vi "xijk_array_to_queue_end.vi"(8 "error in":errorcluster, 9 "timeout in ms (-1)":i32, 10 "array in":T1[](array[typedef]), 11 "queue in":refnum<queue>) -> (0 "error out":errorcluster, 3 "queue out":refnum<queue>)   [LabVIEW 2009]
uses:
  Type Def/event.ctl
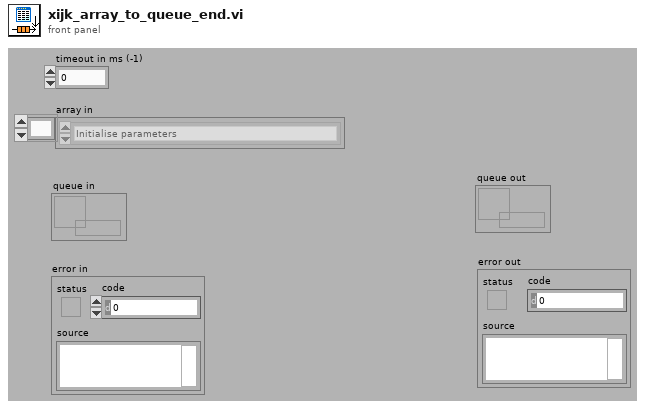
[diagram p1: front panel]
types:
  T1 = typedef "event.ctl" = enum16{"Initialise parameters", "Initialise paths", "Execute", "Hide detector", "Light source selection", "Get example list", "Set Example", "Change portrait / landscape", "Dual band cube", "Save to file", "Load from file", "Set filepaths to boxes", "1 or 2 fluorophore selection", "Update template", "Calculate other values", "Update filter names", "Shutdown", "Shutdown - hard exit", "Search in filters - set parameters", "Search in filters - search", "Search in filters - get xijk", "Search in filters - reget", "Optimize - Sort table", "Get path from search", "Calculate Xijk", "Get spectra from files", "Create graphs", "Reset variables", "Help - open", "Help - close", "Help - next", "Help - previous", "Help - select menu", "Export data"}
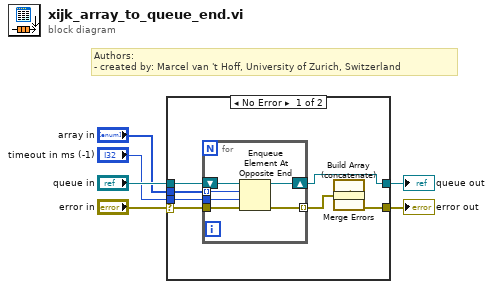
[diagram p0: block diagram]
diagram:
  # "Authors: \n- created by: Marcel van 't Hoff, University of Zurich, Switzerland"
  n1 = case shown="No Error" "error in" {
    selector: "error in" -> [w10 w22]
    tunnel: "queue in" -> [w9 w21]
    tunnel: "array in" -> [w14 _]
    tunnel: [w8 w21] -> w4
    tunnel: [w12 w22] -> w3
    tunnel: "timeout in ms (-1)" -> [w11 _]
    frame #0 {
      n2 = for {
        tunnel: [w20] -> w13 mode=indexing
        tunnel: w10 -> [w19]
        tunnel: w14 -> [w18] mode=indexing
        shift-right: [w15] -> w8
        shift-left: w9 -> [w16]
        tunnel: w11 -> [w17]
        n3 = Enqueue Element At Opposite End(queue=w16, element=w18, timeout in ms (-1)=w17, error in (no error)=w19) -> (queue out=w15:refnum<queue>, error out=w20:errorcluster)  [unwired: 1 out]
      }
      n4 = Build Array (concatenate)(w13) -> (w7:errorcluster[])
      n5 = call <vilib>:"Merge Errors.vi"("error array in"=w7) -> ("error out"=w12:errorcluster)  [unwired: 6 in]
    }
    frame #1 {
    }
  }
  "error out" <- w3
  "queue out" <- w4
